vi "UI_velocity set dialog.vi"(8 "error in (no error)":errorcluster caption="错误输入（无错误）") -> (0 "error out":errorcluster caption="错误输出", 2 "velocity set":T1, 3 "Cancelled?":bool caption="取消？")   [LabVIEW 2017]
doc: "该模板用于创建能够进行事件处理的对话框。"
uses:
  velocity set control.ctl
panel:
  in  "velocity ctl":T1
  in  "旋转电机速度":dbl=1.0
  in  "平移电机速度":dbl=5.0
  in  "Cancel":bool caption="取消"
  in  "OK":bool caption="确定"
  # "Motor velocity set"
  # "Move velocity range: 0-15"
  # "rotation velocity range : 0-45"
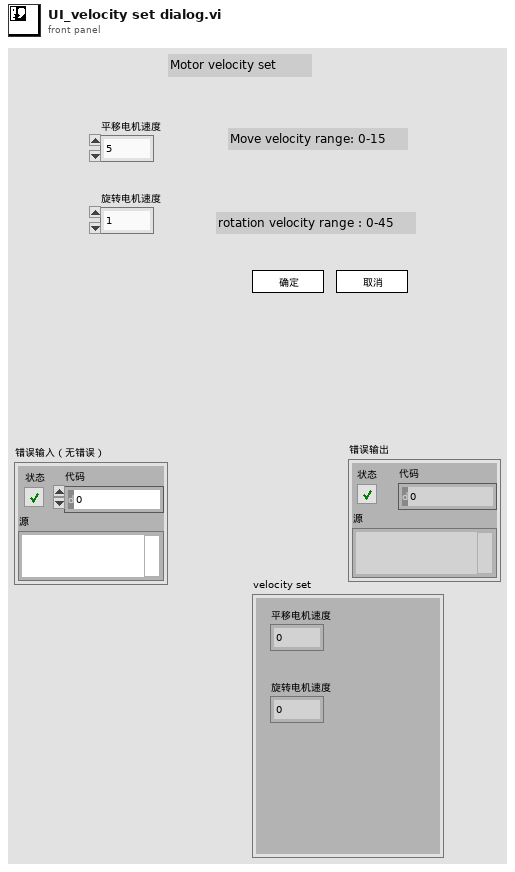
[diagram p1: front panel]
types:
  T1 = typedef "velocity set control.ctl" = cluster{"平移电机速度":dbl, "旋转电机速度":dbl}
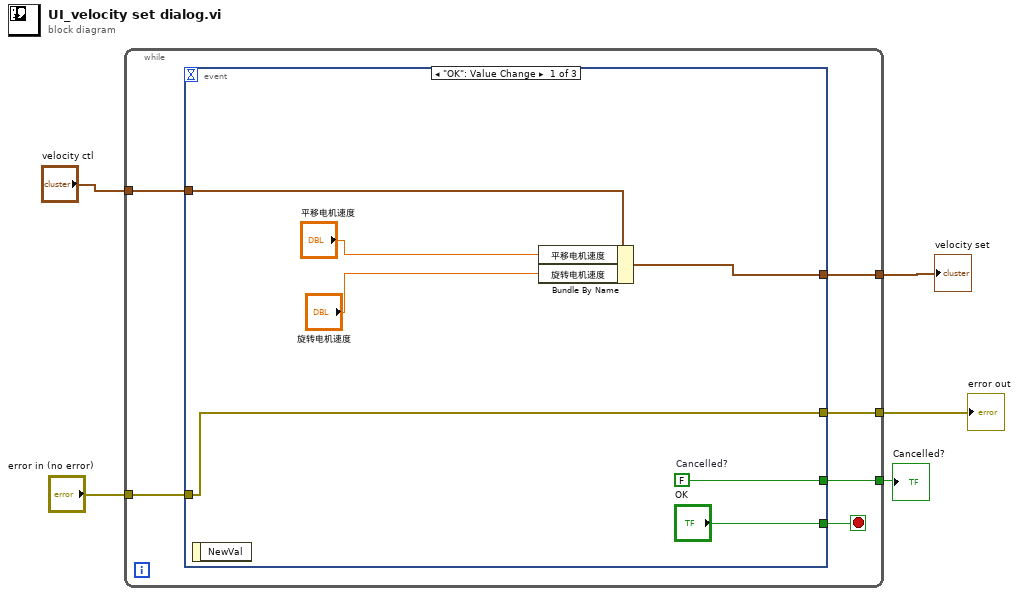
[diagram p0: block diagram]
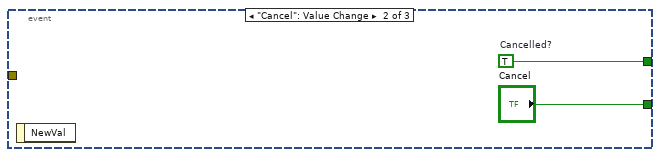
[diagram p2: hidden frame]
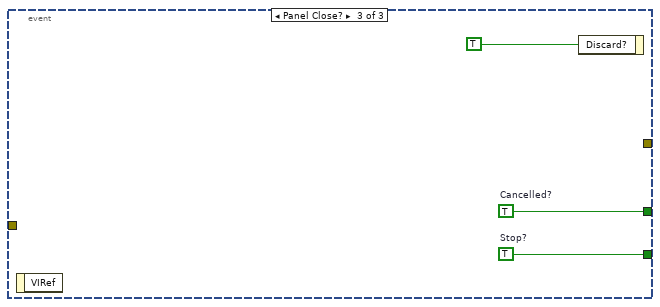
[diagram p3: hidden frame]
diagram:
  n1 = while {
    tunnel: [w10] -> w5
    tunnel: "velocity ctl" -> [w9]
    tunnel: [w8] -> w3
    tunnel: "error in (no error)" -> [w7]
    tunnel: [w6] -> w1
    stop <- w11 stop-if-true
    n2 = event shown="[0] \"OK\": Value Change" {
      selector: _ -> [_ _ _]
      dyn-events: _ -> [_ _ _]
      timeout: _ -> [_ _ _]
      tunnel: ["OK" "Cancel" w22] -> w11
      tunnel: [w18 w20 w21] -> w10
      tunnel: w9 -> [w16 _ _]
      tunnel: [w13 _ _] -> w8
      tunnel: w7 -> [w12 _ _]
      tunnel: [w12 _ _] -> w6
      event "OK": Value Change {
        w18 = FALSE  # Cancelled?
        n3 = event-data() -> ()  [unwired: 1 in, 1 out]
        n4 = Bundle By Name(cluster=w16, "平移电机速度"="平移电机速度", "旋转电机速度"="旋转电机速度") -> (w13:T1)
      }
      event "Cancel": Value Change {
        w20 = TRUE  # Cancelled?
        n5 = event-data() -> ()  [unwired: 1 in, 1 out]
      }
      event Panel Close? {
        w21 = TRUE  # Cancelled?
        w22 = TRUE  # Stop?
        n6 = event-data() -> ()  [unwired: 1 in, 1 out]
        n7 = event-data("Discard?"=TRUE) -> ()  [unwired: 1 in, 1 out]
      }
    }
  }
  "Cancelled?" <- w5
  "velocity set" <- w3
  "error out" <- w1
